vi "PCI-6602 Hardware-Timed Pulse Delay.vi"() -> ()   [LabVIEW 2011]
uses:
  <vilib>/DAQmx/create/channels.llb/DAQmx Create Channel (CO-Pulse Generation-Ticks).vi
  <vilib>/DAQmx/configure/timing.llb/DAQmx Timing (Implicit).vi
  <vilib>/DAQmx/configure/trigger.llb/DAQmx Start Trigger (Digital Edge).vi
  C:/Program Files (x86)/National Instruments/LabVIEW 2011/resource/objmgr/daqmx.rc
panel:
  in  "High Ticks":u32=5
  in  "Low Ticks (Number of Ticks to Wait)":u32=36
  in  "Trigger Source":tag="/PXI1Slot12/PFI1"
  in  "Encoder Signal Input":tag="/PXI1Slot12/PFI0"
  in  "Counter":tag="PXI1Slot12/ctr0"
  in  "Stop":bool
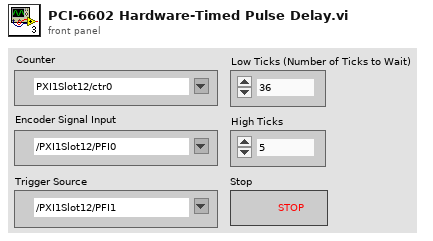
[diagram p1: front panel]
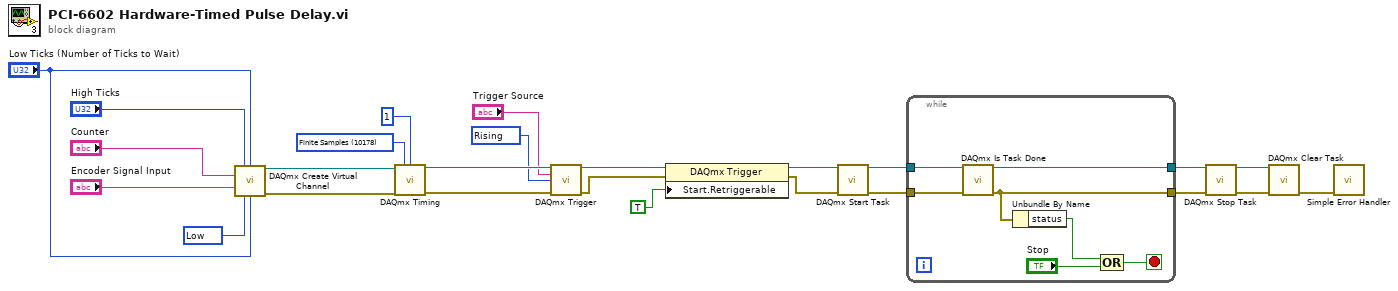
[diagram p0: block diagram]
diagram:
  w4 = 10280 items=["Rising"=10280, "Falling"=10171] ("edge")
  w23 = 10214 items=["High"=10192, "Low"=10214] ("idle state")
  w25 = 10178 items=["Finite Samples"=10178, "Continuous Samples"=10123, "Hardware Timed Single Point"=12522] ("sample mode")
  n1 = call-poly <vilib>:"DAQmx Create Virtual Channel.vi"("high ticks"="High Ticks", "low ticks"="Low Ticks (Number of Ticks to Wait)", "counter"="Counter", "source of ticks"="Encoder Signal Input", "idle state"=w23, "initial delay"="Low Ticks (Number of Ticks to Wait)") -> ("task out"=w22:refnum<k21>, "error out"=w21:errorcluster)  [unwired: 8 in]
  n2 = call-poly <vilib>:"DAQmx Timing.vi"("task/channels in"=w22, "sample mode"=w25, "samples per channel"=1, "error in"=w21) -> ("task out"=w19:refnum<k21>, "error out"=w18:errorcluster)  [unwired: 10 in]
  n3 = call-poly <vilib>:"DAQmx Trigger.vi"("task/channels in"=w19, "source"="Trigger Source", "edge"=w4, "error in"=w18) -> ("task out"=w17:refnum<k21>, "error out"=w16:errorcluster)  [unwired: 10 in]
  n4 = property class="DAQmx Trigger"(reference=w17, error in=w16, "Start.Retriggerable"=TRUE) -> (reference out=w15:refnum<k21>, error out=w14:errorcluster)
  n5 = call <vilib>:"DAQmx Start Task.vi"("task/channels in"=w15, "error in"=w14) -> ("task out"=w13:refnum<k21>, "error out"=w12:errorcluster)  [unwired: 12 in]
  n6 = while {
    tunnel: w13 -> [w32]
    tunnel: w12 -> [w31]
    tunnel: [w30] -> w10
    tunnel: [w29] -> w11
    stop <- w28 stop-if-true
    n7 = call <vilib>:"DAQmx Is Task Done.vi"("task/channels in"=w32, "error in"=w31) -> ("task out"=w29:refnum<k21>, "error out"=w30:errorcluster)  [unwired: 11 in, 1 out]
    n8 = Unbundle By Name(w30) -> ("status"=w26:bool)
    n9 = Compound Arithmetic op=OR(w26, "Stop") -> (w28:bool)
  }
  n10 = call <vilib>:"DAQmx Stop Task.vi"("task/channels in"=w11, "error in"=w10) -> ("task out"=w9:refnum<k21>, "error out"=w8:errorcluster)  [unwired: 12 in]
  n11 = call <vilib>:"DAQmx Clear Task.vi"("task in"=w9, "error in"=w8) -> ("error out"=w2:errorcluster)  [unwired: 13 in]
  n12 = call <vilib>:"Simple Error Handler.vi"("error in (no error)"=w2) -> ()  [unwired: 4 in, 5 out]
